vi "toWhichMonth.vi"(8 "error in (no error)":errorcluster, 11 "Variant":variant) -> (0 "error out":errorcluster, 3 "WhichMonth.lvclass":refnum<class "WhichMonth.lvclass">)   [LabVIEW 2018, in "Account History.lvclass"]
uses:
  Account History.lvclass
  WhichMonth/WhichMonth.lvclass
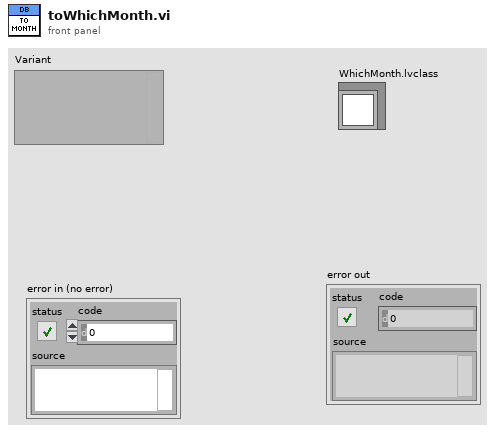
[diagram p1: front panel]
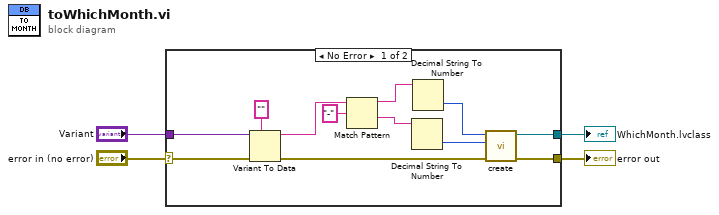
[diagram p0: block diagram]
diagram:
  n1 = case shown="No Error" "error in (no error)" {
    selector: "error in (no error)" -> [w15 w17]
    tunnel: "Variant" -> [w16 _]
    tunnel: [w14 _] -> w2
    tunnel: [w13 w17] -> w1
    frame No Error {
      n2 = Variant To Data(error in=w15, type="", Variant=w16) -> (data=w11:string, error out=w5:errorcluster)
      n3 = Match Pattern(string=w11, regular expression="-") -> (before substring=w9:string, after substring=w8:string)  [unwired: 1 in, 2 out]
      n4 = Decimal String To Number(string=w8) -> (number=w6:i32)  [unwired: 2 in, 1 out]
      n5 = Decimal String To Number(string=w9) -> (number=w7:i32)  [unwired: 2 in, 1 out]
      n6 = call "create.vi"("error in (no error)"=w5, "Month"=w6, "Year"=w7) -> ("error out"=w13:errorcluster, "WhichMonth out"=w14:refnum<class "WhichMonth.lvclass">)  [unwired: 7 in]
    }
    frame Error {
    }
  }
  "WhichMonth.lvclass" <- w2
  "error out" <- w1
